vi "WPI_IMU_ADIS16448_ZeroCorrection.vi"(3 "Z In":dbl, 4 "Y In":dbl, 5 "X In":dbl) -> (0 "Z Out":dbl, 1 "Y Out":dbl, 2 "X Out":dbl)   [LabVIEW 2015, in "Apple Pi Gyro Library.lvlib" / "FRC_ADIS16448_IMU.lvlib"]
uses:
  FRC_ADIS16448_IMU.lvlib
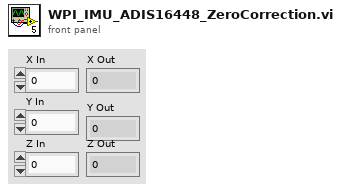
[diagram p1: front panel]
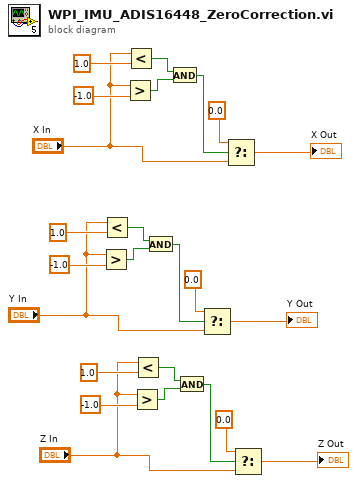
[diagram p0: block diagram]
diagram:
  n1 = Greater?(x="Y In", y=-1.0) -> (0:w13:bool)
  n2 = Less?(x="Y In", y=1.0) -> (x < y?=w12:bool)
  n3 = Greater?(x="X In", y=-1.0) -> (0:w21:bool)
  n4 = Less?(x="X In", y=1.0) -> (x < y?=w20:bool)
  n5 = Greater?(x="Z In", y=-1.0) -> (0:w5:bool)
  n6 = Less?(x="Z In", y=1.0) -> (x < y?=w4:bool)
  n7 = And(x=w12, y=w13) -> (x .and. y?=w11:bool)
  n8 = And(x=w20, y=w21) -> (x .and. y?=w19:bool)
  n9 = And(x=w4, y=w5) -> (x .and. y?=w3:bool)
  n10 = Select(t=0.0, s=w11, f="Y In") -> (s? t:f=→"Y Out":dbl)
  n11 = Select(t=0.0, s=w19, f="X In") -> (s? t:f=→"X Out":dbl)
  n12 = Select(t=0.0, s=w3, f="Z In") -> (s? t:f=→"Z Out":dbl)
